vi "ManipIntake.vi"(2 "Reinit":bool, 3 "Instruction String":string) -> (0 "Error Out":errorcluster, 1 "Advance Trigger":bool)   [LabVIEW 2019]
doc: "Toggles the intake deployment state.\n\nParameters: None"
uses:
  dsinstructions.vi
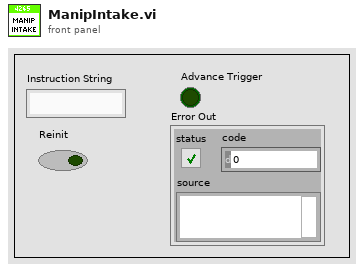
[diagram p1: front panel]
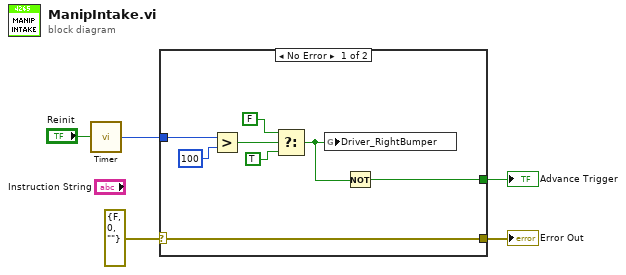
[diagram p0: block diagram]
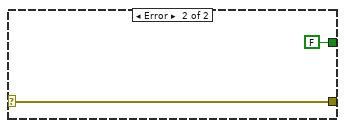
[diagram p2: hidden frame]
diagram:
  n1 = call "Timer.vi"("Reset Timer"="Reinit") -> ("Time (ms)"=w2:u32)
  n2 = case shown="No Error" errorcluster {"status"=FALSE, "code"=0, "source"=""} ("error constant") {
    selector: errorcluster {"status"=FALSE, "code"=0, "source"=""} ("error constant") -> [w7 w15]
    tunnel: [w8 FALSE] -> w5
    tunnel: [w7 w15] -> w3
    tunnel: w2 -> [w6 _]
    frame No Error {
      n3 = Greater?(x=w6, y=u32 100) -> (0:w12:bool)
      n4 = Select(t=FALSE, s=w12, f=TRUE ("Driver_RightBumper")) -> (s? t:f=w9:bool)
      n5 = global write "dsinstructions.vi" "Driver_RightBumper"(w9) -> ()
      n6 = Not(x=w9) -> (.not. x?=w8:bool)
    }
    frame Error {
    }
  }
  "Advance Trigger" <- w5
  "Error Out" <- w3
